vi "Python Test.vi"   [LabVIEW 2017]
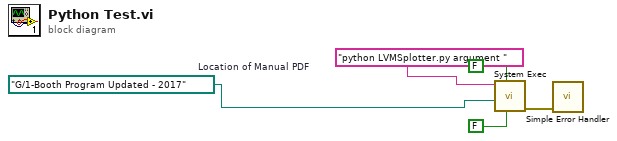
[diagram p0: block diagram]
diagram:
  w2 = path "G:/1-Booth Program Updated - 2017"  # Location of Manual PDF
  n1 = call <vilib>:"System Exec.vi"("run minimized? (F)"=FALSE, "wait until completion? (T)"=FALSE ("wait until ? (T)"), "working directory"=w2, "command line"="python LVMSplotter.py argument ") -> ("error out"=w3:errorcluster)  [unwired: 2 in, 5 out]
  n2 = call <vilib>:"Simple Error Handler.vi"("error in (no error)"=w3) -> ()  [unwired: 4 in, 5 out]
